vi "test.vi"() -> ()   [LabVIEW 2017]
uses:
  libMPSSE.lvlib
panel:
  out "sizeTransfered":u32
  in  "options read":T1={"Start bit"=TRUE, "Stop bit"=TRUE, "Acknowledge bit"=TRUE, "Reserved bit"=FALSE, "Multi byte I2C"=FALSE, "Multi bit I2C"=FALSE, "Ignore address"=FALSE, "Reserved bit 2"=FALSE}
  in  "Data to write":u8[](array[numeric])=[0, 0] format="%02x"
  in  "Config":T2={"ClockRate"=100000, "LatencyTimer"=1, "Disable 3 phase clocking"=FALSE, "Disable drive only 0"=FALSE} {"ClockRate" items=["I2C_CLOCK_STANDARD_MODE"=100000, "I2C_CLOCK_FAST_MODE"=400000, "I2C_CLOCK_FAST_MODE_PLUS"=1000000, "I2C_CLOCK_HIGH_SPEED_MODE"=3400000]}
  out "Data read":u8[](array[numeric]) format="%.0x"
  in  "options write":T1={"Start bit"=TRUE, "Stop bit"=FALSE, "Acknowledge bit"=TRUE, "Reserved bit"=FALSE, "Multi byte I2C"=FALSE, "Multi bit I2C"=FALSE, "Ignore address"=FALSE, "Reserved bit 2"=FALSE}
  in  "sizeToTransfer":u32=1
  in  "deviceAddress":u32=80 format="%.0b"
  out "numChannels out":u32
  out "error out":errorcluster
  # "This VI read an address of an EEPROM on I2C"
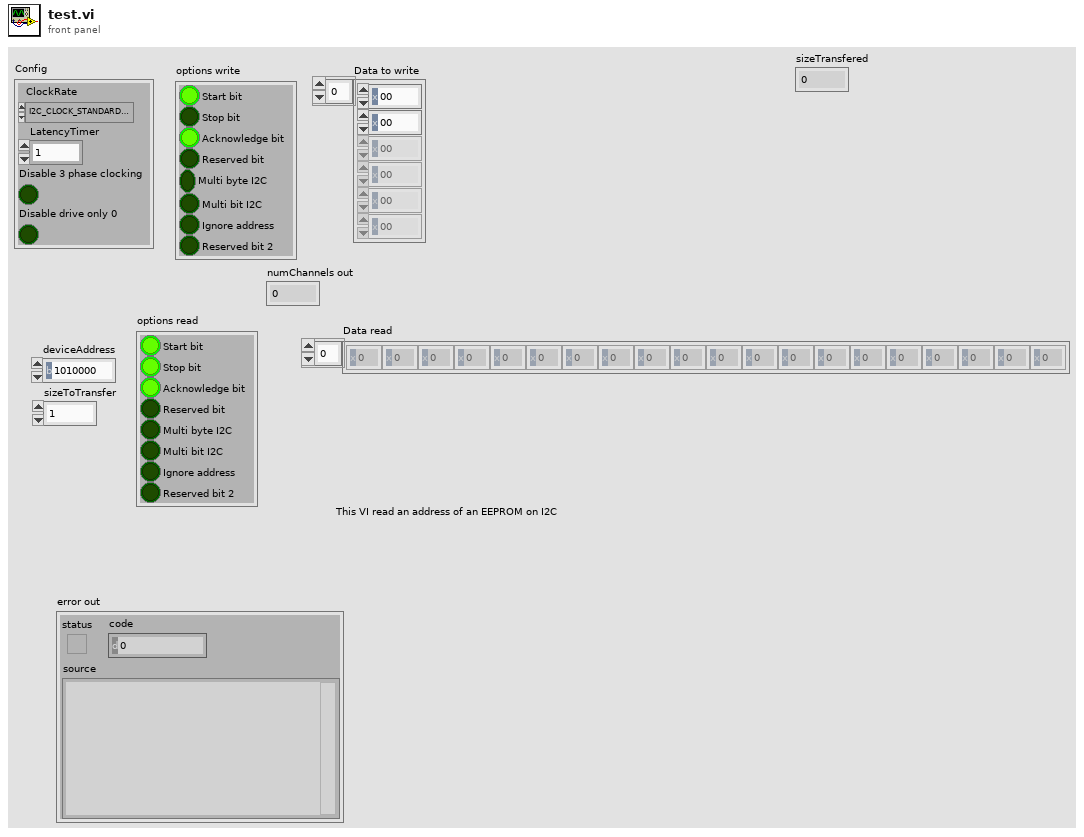
[diagram p1: front panel]
types:
  T1 = cluster{"Start bit":bool, "Stop bit":bool, "Acknowledge bit":bool, "Reserved bit":bool, "Multi byte I2C":bool, "Multi bit I2C":bool, "Ignore address":bool, "Reserved bit 2":bool}
  T2 = cluster{"ClockRate":u32, "LatencyTimer":u8, "Disable 3 phase clocking":bool, "Disable drive only 0":bool}
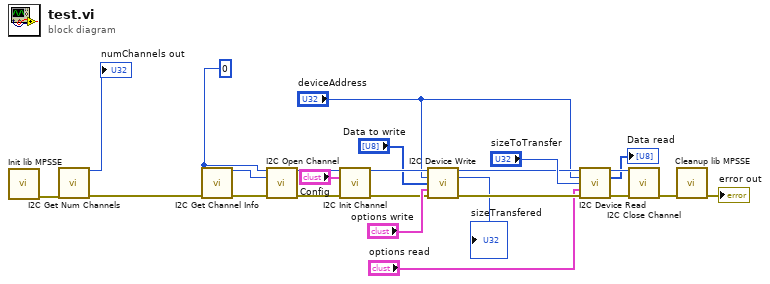
[diagram p0: block diagram]
diagram:
  w18 = u32 0 ("index")
  n1 = call "Init lib MPSSE.vi"() -> ("error out"=w24:errorcluster)  [unwired: 15 in]
  n2 = call "I2C Get Num Channels.vi"("error in (no error)"=w24) -> ("numChannels out"=→"numChannels out":u32, "error out"=w20:errorcluster)  [unwired: 13 in]
  n3 = call "I2C Get Channel Info.vi"("index"=w18, "error in (no error)"=w20) -> ("ftHandle"=w14:u32, "error out"=w19:errorcluster)  [unwired: 6 in, 6 out]
  n4 = call "I2C Open Channel.vi"("handle"=w18, "index"=w14, "error in (no error)"=w19) -> ("handle out"=w16:u32, "error out"=w15:errorcluster)  [unwired: 11 in]
  n5 = call "I2C Init Channel.vi"("handle"=w16, "Config"="Config", "error in (no error)"=w15) -> ("handle out"=w9:u32, "error out"=w8:errorcluster)  [unwired: 11 in]
  n6 = call "I2C Device Write.vi"("handle"=w9, "deviceAddress"="deviceAddress", "Data to write"="Data to write", "options"="options write", "error in (no error)"=w8) -> ("handle out"=w11:u32, "sizeTransfered"=→"sizeTransfered":u32, "error out"=w12:errorcluster)  [unwired: 8 in]
  n7 = call "I2C Device Read.vi"("handle"=w11, "Slave device address"="deviceAddress", "Size to transfer"="sizeToTransfer", "options"="options read", "error in (no error)"=w12) -> ("handle out"=w6:u32, "Data read"=→"Data read":u8[], "error out"=w7:errorcluster)  [unwired: 8 in]
  n8 = call "I2C Close Channel.vi"("handle"=w6, "error in (no error)"=w7) -> ("error out"=w21:errorcluster)  [unwired: 13 in]
  n9 = call "Cleanup lib MPSSE.vi"("error in (no error)"=w21) -> ("error out"=→"error out":errorcluster)  [unwired: 14 in]
